vi "Mérési adatok FIFO-ba.vi"(8 "error in":errorcluster, 10 "Bemenõ adatok":dbl[][](array[numeric]) format="%0.2f", 11 "Analog data":T1) -> (0 "error out":errorcluster, 3 "Analog data out":T1)   [LabVIEW 2014]
uses:
  Analog data.ctl
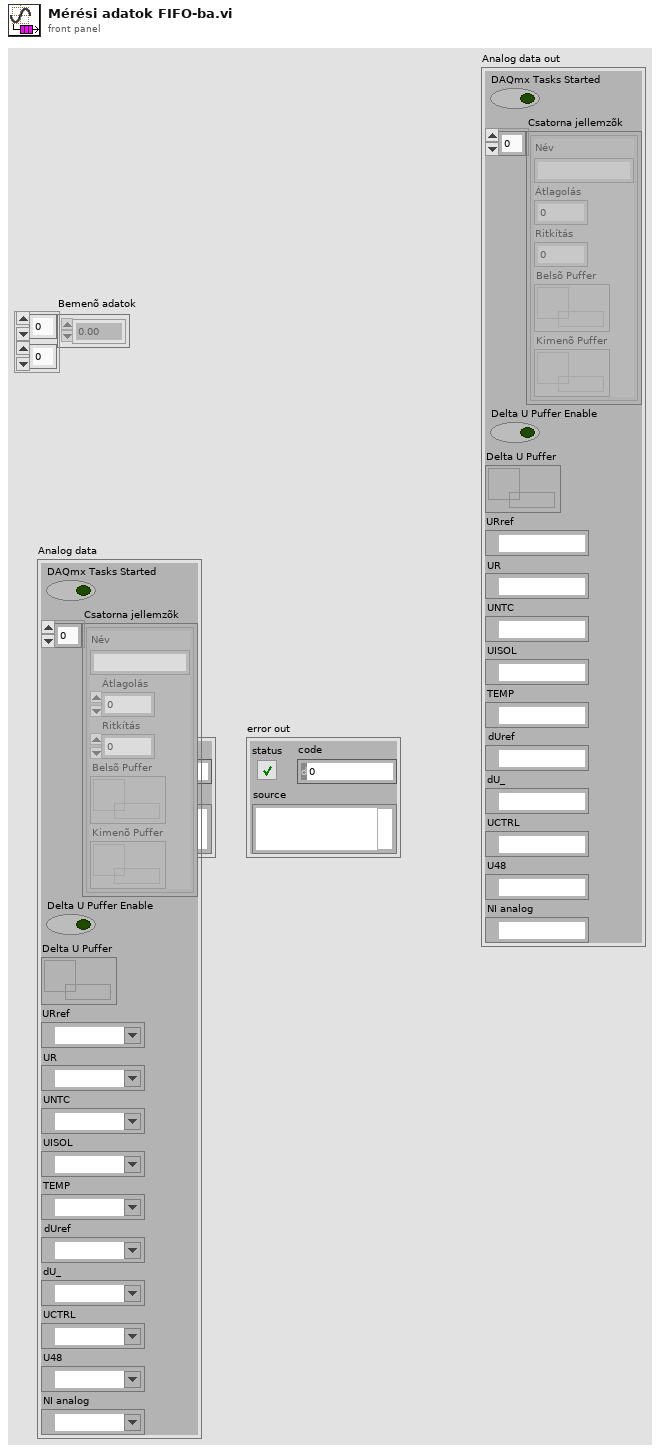
[diagram p1: front panel]
types:
  T1 = typedef "Analog data.ctl" = cluster{"DAQmx Tasks Started":bool, "Csatorna jellemzõk":T2[], "Delta U Puffer Enable":bool, "Delta U Puffer":refnum<queue>, "URref":refnum<k21>, "UR":refnum<k21>, "UNTC":refnum<k21>, "UISOL":refnum<k21>, "TEMP":refnum<k21>, "dUref":refnum<k21>, "dU_":refnum<k21>, "UCTRL":refnum<k21>, "U48":refnum<k21>, "NI analog":refnum<k21>}
  T2 = typedef "Csatorna jellemzõk.ctl" = cluster{"Név":string, "Átlagolás":i32, "Ritkítás":i32, "Belsõ Puffer":refnum<queue>, "Kimenõ Puffer":refnum<queue>}
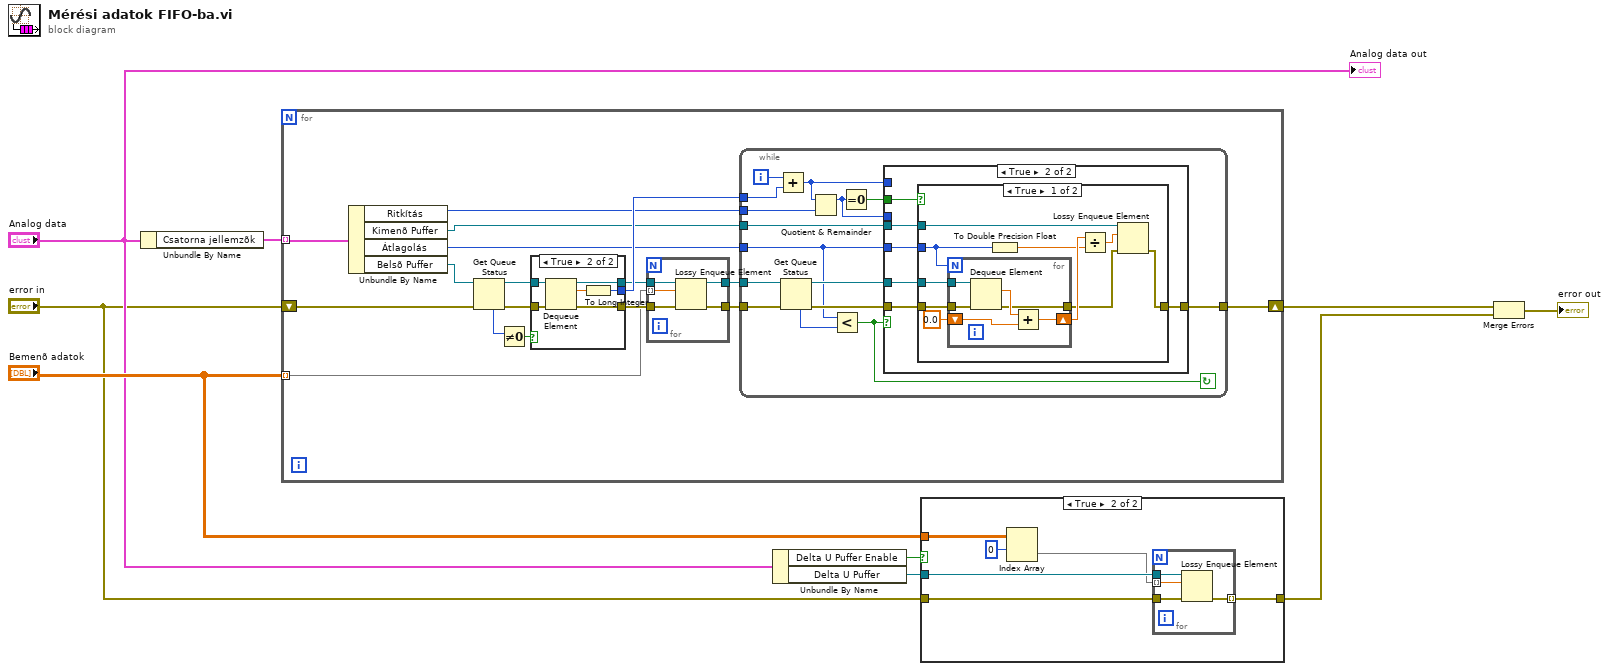
[diagram p0: block diagram]
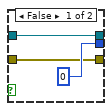
[diagram p3: hidden frame]
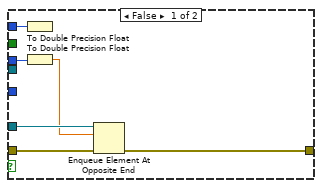
[diagram p4: hidden frame]
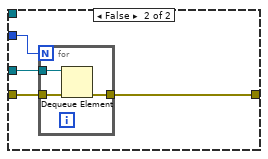
[diagram p5: hidden frame]
diagram:
  n1 = Unbundle By Name("Analog data") -> ("Csatorna jellemzõk"=w9:T2[])
  n2 = for {
    tunnel: w9 -> [w12] mode=indexing
    tunnel: "Bemenõ adatok" -> [w11] mode=indexing
    shift-right: [w19] -> w2
    shift-left: "error in" -> [w10]
    n3 = Unbundle By Name(w12) -> ("Ritkítás"=w16:i32, "Kimenõ Puffer"=w15:refnum<queue>, "Átlagolás"=w14:i32, "Belsõ Puffer"=w13:refnum<queue>)
    n4 = Get Queue Status(queue=w13, error in (no error)=w10) -> (queue out=w20:refnum<queue>, error out=w22:errorcluster, # elements in queue=w23:i32)  [unwired: 1 in, 5 out]
    n5 = Not Equal To 0?(x=w23) -> (x != 0?=w24:bool)
    n6 = case shown="True" w24 {
      tunnel: w22 -> [w28 w34]
      tunnel: w20 -> [w27 w35]
      tunnel: [w27 w33] -> w21
      tunnel: [0 w31] -> w25
      tunnel: [w28 w30] -> w26
      frame False {
      }
      frame True {
        n7 = Dequeue Element(queue=w35, error in (no error)=w34) -> (queue out=w33:refnum<queue>, element=w32:dbl, error out=w30:errorcluster)  [unwired: 1 in, 1 out]
        n8 = To Long Integer(number=w32) -> (32bit integer=w31:i32)
      }
    }
    n9 = for {
      tunnel: w11 -> [w90] mode=indexing
      tunnel: w21 -> [w89]
      tunnel: [w88] -> w17
      tunnel: [w87] -> w18
      tunnel: w26 -> [w86]
      n10 = Lossy Enqueue Element(queue=w89, element=w90, error in (no error)=w86) -> (queue out=w87:refnum<queue>, error out=w88:errorcluster)  [unwired: 2 out]
    }
    n11 = while {
      tunnel: w18 -> [w50]
      tunnel: w15 -> [w47]
      tunnel: w17 -> [w45]
      tunnel: w14 -> [w43]
      tunnel: w16 -> [w41]
      tunnel: [w40] -> w19
      tunnel: w25 -> [w38]
      i -> [w39]
      stop <- w46 continue-if-true
      n12 = Add(x=w39, y=w38) -> (x+y=w37:i32)
      n13 = Get Queue Status(queue=w50, error in (no error)=w45) -> (queue out=w48:refnum<queue>, error out=w44:errorcluster, # elements in queue=w49:i32)  [unwired: 1 in, 5 out]
      n14 = Quotient & Remainder(x=w37, y=w41) -> (x-y*floor(x/y)=w36:i32)  [unwired: 1 out]
      n15 = Less?(x=w43, y=w49) -> (x < y?=w46:bool)
      n16 = Equal To 0?(x=w36) -> (x = 0?=w42:bool)
      n17 = case shown="True" w46 {
        tunnel: w48 -> [w54 w62]
        tunnel: w47 -> [_ w61]
        tunnel: w43 -> [_ w59]
        tunnel: w44 -> [w56 w60]
        tunnel: w42 -> [_ w58]
        tunnel: [w55 w57] -> w40
        tunnel: w37 -> [w53 _]
        tunnel: w36 -> [w52 _]
        frame False {
          n18 = To Double Precision Float(number=w53) -> ()  [unwired: 1 out]
          n19 = To Double Precision Float(number=w52) -> (double precision float=w51:dbl)
          n20 = Enqueue Element At Opposite End(queue=w54, element=w51, error in (no error)=w56) -> (error out=w55:errorcluster)  [unwired: 1 in, 2 out]
        }
        frame True {
          n21 = case shown="True" w58 {
            tunnel: w62 -> [w72 w82]
            tunnel: w61 -> [w69 _]
            tunnel: w60 -> [w68 w81]
            tunnel: w59 -> [w67 w80]
            tunnel: [w63 w79] -> w57
            frame True {
              n22 = for {
                N: w67 -> [_]
                tunnel: w72 -> [w78]
                shift-right: [w75] -> w70
                shift-left: 0.0 -> [w76]
                tunnel: w68 -> [w74]
                tunnel: [w73] -> w64
                n23 = Dequeue Element(queue=w78, error in (no error)=w74) -> (element=w77:dbl, error out=w73:errorcluster)  [unwired: 1 in, 2 out]
                n24 = Add(x=w77, y=w76) -> (x+y=w75:dbl)
              }
              n25 = To Double Precision Float(number=w67) -> (double precision float=w65:dbl)
              n26 = Divide(x=w70, y=w65) -> (x/y=w66:dbl)
              n27 = Lossy Enqueue Element(queue=w69, element=w66, error in (no error)=w64) -> (error out=w63:errorcluster)  [unwired: 3 out]
            }
            frame False {
              n28 = for {
                N: w80 -> [_]
                tunnel: w82 -> [w85]
                tunnel: w81 -> [w84]
                tunnel: [w83] -> w79
                n29 = Dequeue Element(queue=w85, error in (no error)=w84) -> (error out=w83:errorcluster)  [unwired: 1 in, 3 out]
              }
            }
          }
        }
      }
    }
  }
  n30 = Unbundle By Name("Analog data") -> ("Delta U Puffer Enable"=w5:bool, "Delta U Puffer"=w6:refnum<queue>)
  n31 = case shown="True" w5 {
    tunnel: "Bemenõ adatok" -> [_ w96]
    tunnel: w6 -> [_ w94]
    tunnel: "error in" -> [_ w92]
    tunnel: [_ w91] -> w1
    frame False {
    }
    frame True {
      n32 = Index Array(array=w96, index (row)=0) -> (element=w93:dbl[])  [unwired: 1 in]
      n33 = for {
        tunnel: w94 -> [w100]
        tunnel: w93 -> [w99] mode=indexing
        tunnel: w92 -> [w98]
        tunnel: [w97] -> w91 mode=indexing
        n34 = Lossy Enqueue Element(queue=w100, element=w99, error in (no error)=w98) -> (error out=w97:errorcluster)  [unwired: 3 out]
      }
    }
  }
  n35 = Merge Errors(w2, w1) -> (→"error out":errorcluster)
  "Analog data out" <- "Analog data"
